vi "Spectral Data Organize (SubVI).vi"(0 "Measurement Cluster IN":T2, 2 "Data Array IN":dbl[](array[numeric]), 3 "Ref Lamp Mode":T1(radio), 5 "Collect Background":bool, 9 "Write Spectral Data IN":bool, 11 "Take Ref Lamp":bool, 13 "Ref Lamp at Flame Loc File":path=path "C:/Users/bedickc/Documents/_MHD/K Spectroscopy (Ocean Optics Spectrometer)/20171005_HR4000_KOptics_Calib/Lamp_At_Flame_Location_ND10Corr_HR4000_LabviewWavelengths.csv", 15 "Integration Time (ms)":dbl format="%#_13g", 17 "ON/OFF IN":bool) -> (19 "ON/OFF OUT":bool, 20 "Measurement Cluster OUT":T2, 25 "Write Spectral Data OUT":bool, 26 "Reset ON/OFF":bool)   [LabVIEW 2015]
uses:
  Measurement Cluster.ctl
  <vilib>/Utility/file.llb/Read Delimited Spreadsheet (DBL).vi
  <vilib>/Utility/file.llb/Write Delimited Spreadsheet (DBL).vi
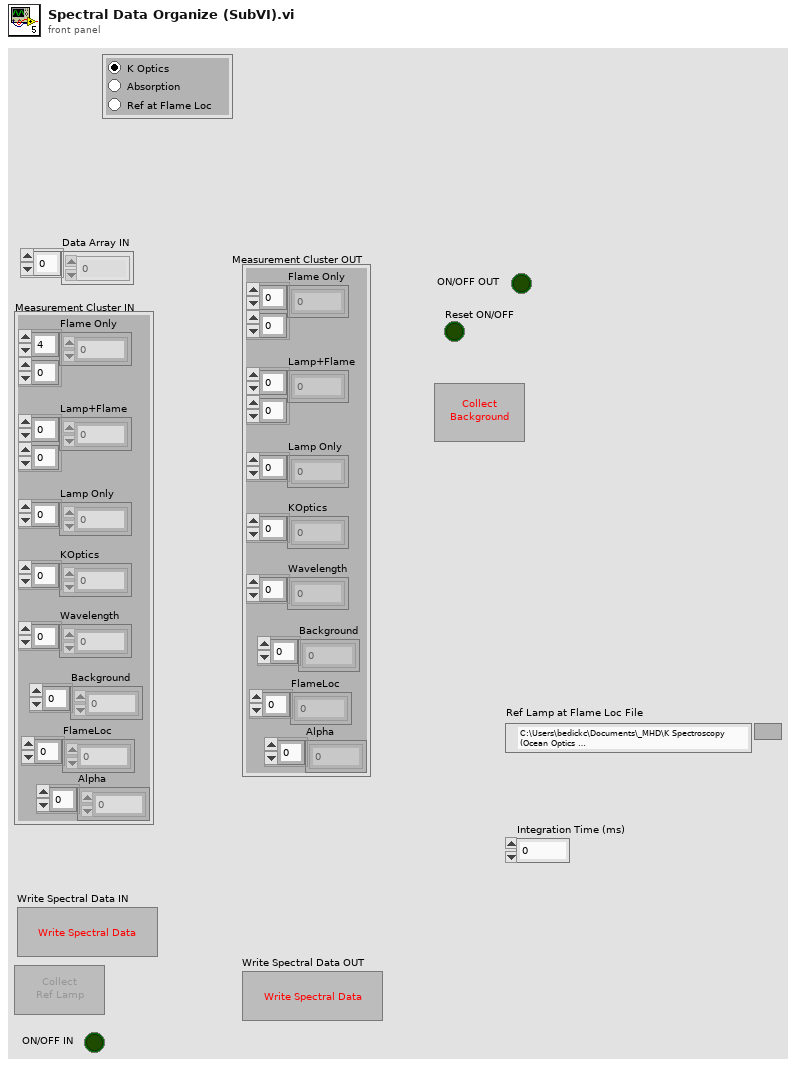
[diagram p1: front panel]
types:
  T1 = enum32{"K Optics", "Absorption", "Ref at Flame Loc"}
  T2 = typedef "Measurement Cluster.ctl" = cluster{"Flame Only":dbl[][], "Lamp+Flame":dbl[][], "Lamp Only":dbl[], "KOptics":dbl[], "Wavelength":dbl[], "Background":dbl[], "FlameLoc":dbl[], "Alpha":dbl[]}
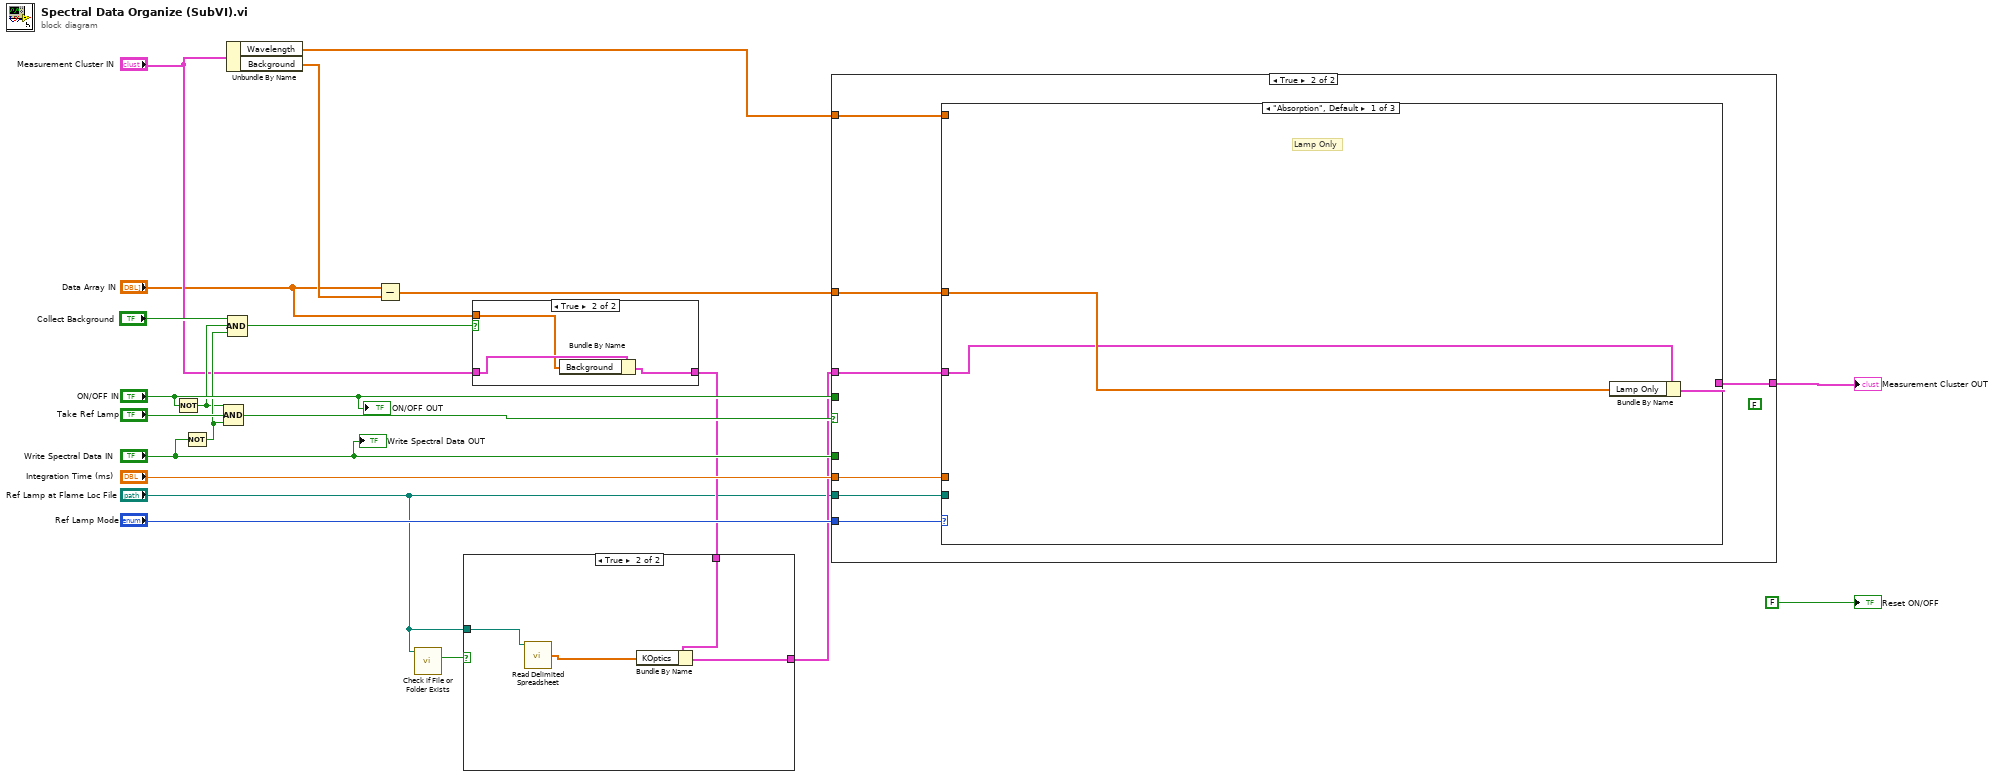
[diagram p0: block diagram]
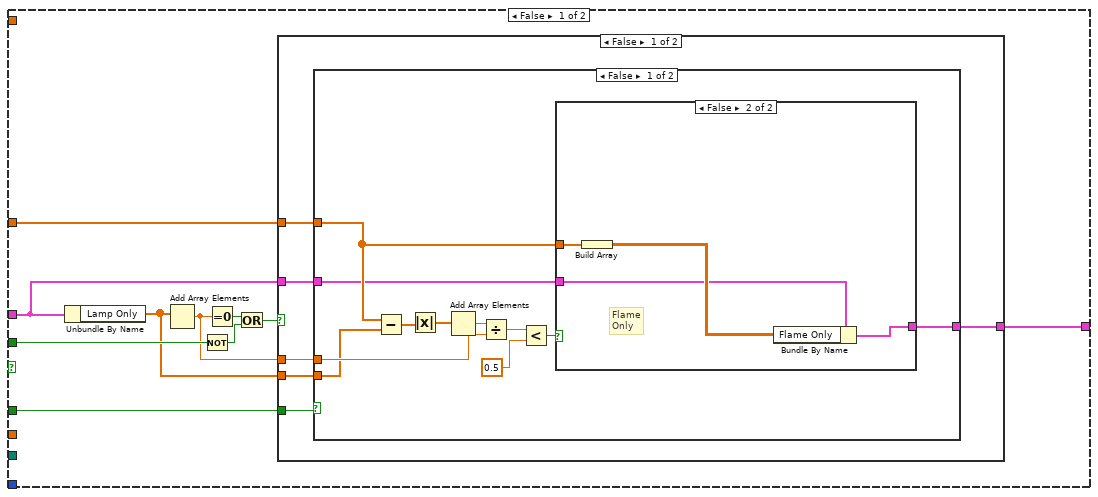
[diagram p3: hidden frame]
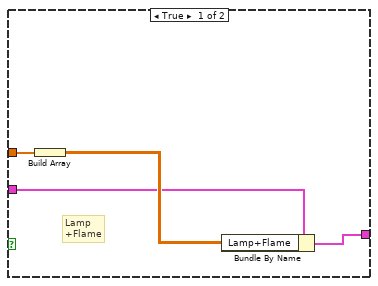
[diagram p4: hidden frame]
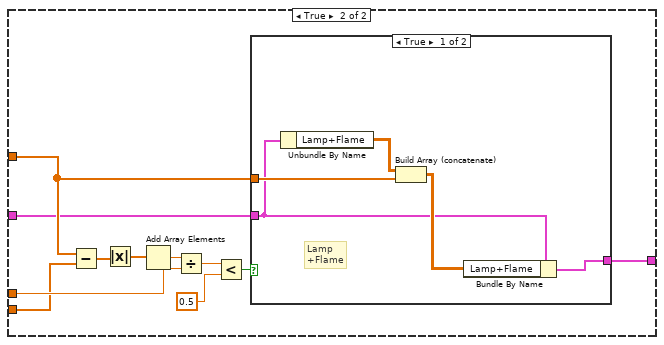
[diagram p5: hidden frame]
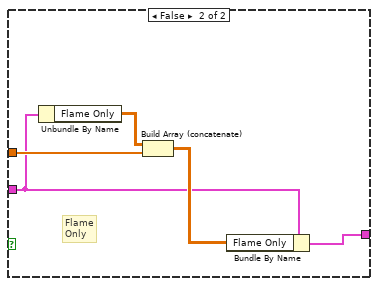
[diagram p6: hidden frame]
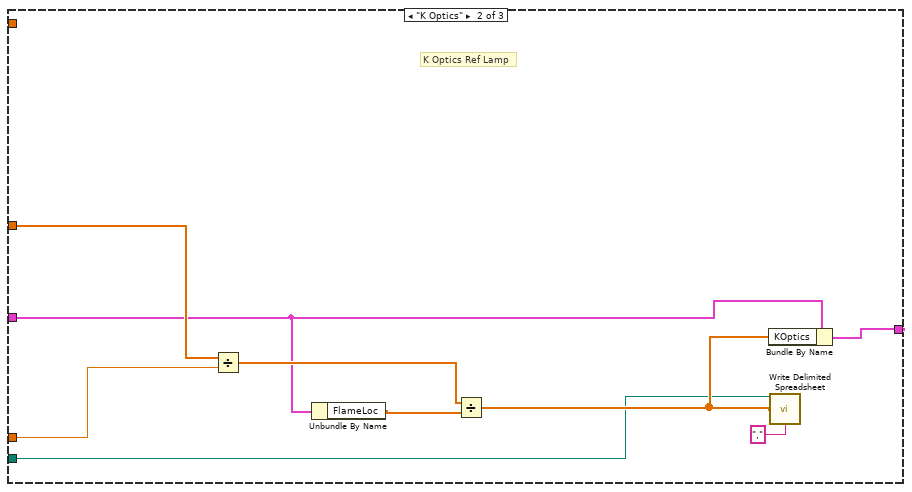
[diagram p8: hidden frame]
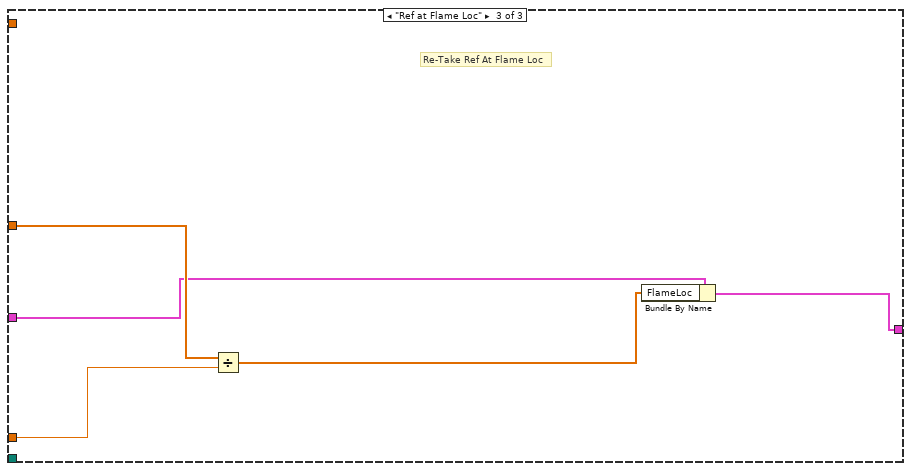
[diagram p9: hidden frame]
diagram:
  n1 = Not(x="ON/OFF IN") -> (.not. x?=w8:bool)
  n2 = Not(x="Write Spectral Data IN") -> (.not. x?=w9:bool)
  n3 = Compound Arithmetic op=AND(w8, "Take Ref Lamp", w9) -> (w20:bool)
  n4 = Unbundle By Name("Measurement Cluster IN") -> ("Wavelength"=w18:dbl[], "Background"=w12:dbl[])
  n5 = Compound Arithmetic op=AND("Collect Background", w8, w9) -> (w6:bool)
  n6 = Subtract(x="Data Array IN", y=w12) -> (x-y=w13:dbl[])
  n7 = call <vilib>:"Check if File or Folder Exists.vi"("path"="Ref Lamp at Flame Loc File") -> ("file or folder exists?"=w4:bool)  [unwired: 8 in, 2 out]
  n8 = case shown="True" w6 {
    tunnel: "Measurement Cluster IN" -> [w22 w24]
    tunnel: [w22 w25] -> w3
    tunnel: "Data Array IN" -> [_ w23]
    frame False {
    }
    frame True {
      n9 = Bundle By Name(cluster=w24, "Background"=w23) -> (w25:T2)
    }
  }
  n10 = case shown="True" w4 {
    tunnel: w3 -> [w26 w29]
    tunnel: [w26 w28] -> w2
    tunnel: "Ref Lamp at Flame Loc File" -> [_ w27]
    frame False {
    }
    frame True {
      n11 = call-poly <vilib>:"Read Delimited Spreadsheet.vi"("file path (dialog if empty)"=w27) -> ("first row"=w30:dbl[])  [unwired: 9 in, 5 out]
      n12 = Bundle By Name(cluster=w29, "KOptics"=w30) -> (w28:T2)
    }
  }
  n13 = case shown="True" w20 {
    tunnel: w13 -> [w40 w89]
    tunnel: "Write Spectral Data IN" -> [w39 _]
    tunnel: "ON/OFF IN" -> [w37 _]
    tunnel: "Ref Lamp at Flame Loc File" -> [_ w94]
    tunnel: "Integration Time (ms)" -> [_ w93]
    tunnel: w18 -> [_ w92]
    tunnel: [w33 w91] -> w17
    tunnel: w2 -> [w34 w90]
    tunnel: "Ref Lamp Mode" -> [_ w88]
    frame False {
      n14 = Unbundle By Name(w34) -> ("Lamp Only"=w31:dbl[])
      n15 = Add Array Elements(numeric array=w31) -> (sum=w32:dbl)
      n16 = Not(x=w37) -> (.not. x?=w36:bool)
      n17 = Equal To 0?(x=w32) -> (x = 0?=w38:bool)
      n18 = Or(x=w38, y=w36) -> (x .or. y?=w35:bool)
      n19 = case shown="False" w35 {
        tunnel: w40 -> [w45 _]
        tunnel: w39 -> [w46 _]
        tunnel: w34 -> [w44 w87]
        tunnel: [w43 w87] -> w33
        tunnel: w32 -> [w42 _]
        tunnel: w31 -> [w41 _]
        frame False {
          n20 = case shown="False" w46 {
            tunnel: w45 -> [w51 w70]
            tunnel: w44 -> [w50 w69]
            tunnel: [w49 w68] -> w43
            tunnel: w42 -> [w48 w67]
            tunnel: w41 -> [w47 w66]
            frame False {
              n21 = Subtract(x=w51, y=w47) -> (x-y=w56:dbl[])
              n22 = Absolute Value(x=w56) -> (abs(x)=w57:dbl[])
              n23 = Add Array Elements(numeric array=w57) -> (sum=w54:dbl)
              n24 = Divide(x=w54, y=w48) -> (x/y=w55:dbl)
              n25 = Less?(x=w55, y=0.5) -> (x < y?=w52:bool)
              n26 = case shown="False" w52 {
                tunnel: w51 -> [w61 w65]
                tunnel: w50 -> [w59 w63]
                tunnel: [w58 w62] -> w49
                frame True {
                  # "Lamp\n+Flame"
                  n27 = Build Array(w61) -> (w60:dbl[][])
                  n28 = Bundle By Name(cluster=w59, "Lamp+Flame"=w60) -> (w58:T2)
                }
                frame False {
                  # "Flame\nOnly"
                  n29 = Build Array(w65) -> (w64:dbl[][])
                  n30 = Bundle By Name(cluster=w63, "Flame Only"=w64) -> (w62:T2)
                }
              }
            }
            frame True {
              n31 = Subtract(x=w70, y=w66) -> (x-y=w75:dbl[])
              n32 = Absolute Value(x=w75) -> (abs(x)=w76:dbl[])
              n33 = Add Array Elements(numeric array=w76) -> (sum=w73:dbl)
              n34 = Divide(x=w73, y=w67) -> (x/y=w74:dbl)
              n35 = Less?(x=w74, y=0.5) -> (x < y?=w71:bool)
              n36 = case shown="True" w71 {
                tunnel: w70 -> [w81 w86]
                tunnel: w69 -> [w77 w82]
                tunnel: [w79 w84] -> w68
                frame True {
                  # "Lamp\n+Flame"
                  n37 = Unbundle By Name(w77) -> ("Lamp+Flame"=w78:dbl[][])
                  n38 = Build Array (concatenate)(w78, w81) -> (w80:dbl[][])
                  n39 = Bundle By Name(cluster=w77, "Lamp+Flame"=w80) -> (w79:T2)
                }
                frame False {
                  # "Flame\nOnly"
                  n40 = Unbundle By Name(w82) -> ("Flame Only"=w83:dbl[][])
                  n41 = Build Array (concatenate)(w83, w86) -> (w85:dbl[][])
                  n42 = Bundle By Name(cluster=w82, "Flame Only"=w85) -> (w84:T2)
                }
              }
            }
          }
        }
        frame True {
        }
      }
    }
    frame True {
      (unwired) FALSE
      n43 = case shown="\"Absorption\", Default" w88 {
        tunnel: w94 -> [_ w98 _]
        tunnel: w93 -> [_ w106 w111]
        tunnel: w92 -> [_ _ _]
        tunnel: [w97 w105 w108] -> w91
        tunnel: w90 -> [w95 w101 w109]
        tunnel: w89 -> [w96 w104 w110]
        frame "Absorption", Default {
          # "Lamp Only"
          n44 = Bundle By Name(cluster=w95, "Lamp Only"=w96) -> (w97:T2)
        }
        frame "K Optics" {
          # "K Optics Ref Lamp"
          n45 = Divide(x=w104, y=w106) -> (x/y=w103:dbl[])
          n46 = Unbundle By Name(w101) -> ("FlameLoc"=w102:dbl[])
          n47 = Divide(x=w103, y=w102) -> (x/y=w99:dbl[])
          n48 = Bundle By Name(cluster=w101, "KOptics"=w99) -> (w105:T2)
          n49 = call-poly <vilib>:"Write Delimited Spreadsheet.vi"("file path (dialog if empty)"=w98, "1D data"=w99, "delimiter (\\t)"="," ("delimiter (\\t)")) -> ()  [unwired: 11 in, 2 out]
        }
        frame "Ref at Flame Loc" {
          # "Re-Take Ref At Flame Loc"
          n50 = Divide(x=w110, y=w111) -> (x/y=w107:dbl[])
          n51 = Bundle By Name(cluster=w109, "FlameLoc"=w107) -> (w108:T2)
        }
      }
    }
  }
  "Measurement Cluster OUT" <- w17
  "Write Spectral Data OUT" <- "Write Spectral Data IN"
  "ON/OFF OUT" <- "ON/OFF IN"
  "Reset ON/OFF" <- FALSE
